vi "Ch_data_title_pattern (SubVI).vi"(9 "Единица измерений":string) -> (0 "error out":errorcluster, 2 "Path":path, 3 "Byte Stream File out":refnum<file>)   [LabVIEW 2015]
panel:
  in  "error in":errorcluster
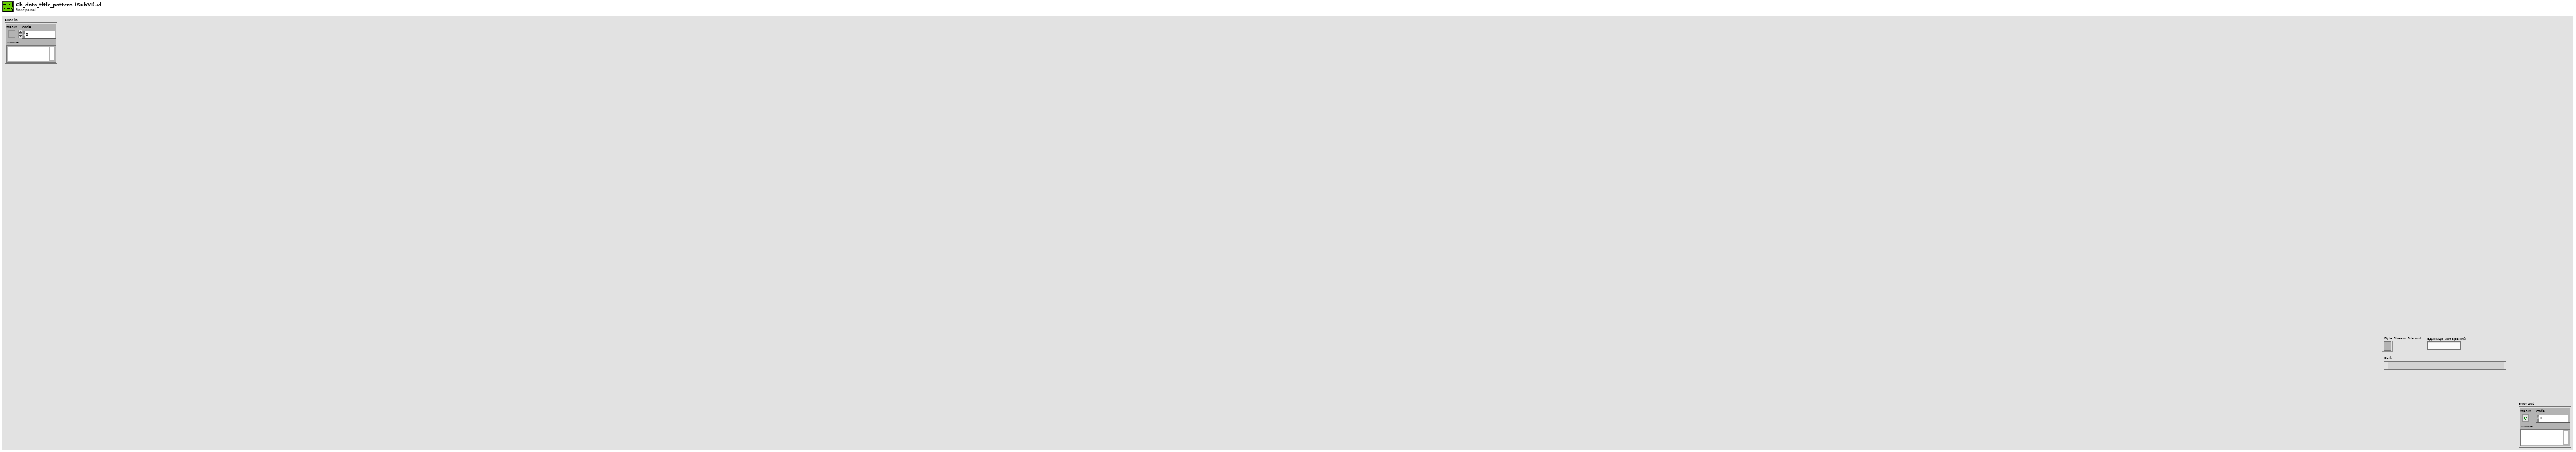
[diagram p1: front panel]
types:
  T1 = enum16{"open", "replace", "create", "open or create", "replace or create", "replace or create with confirmation"}
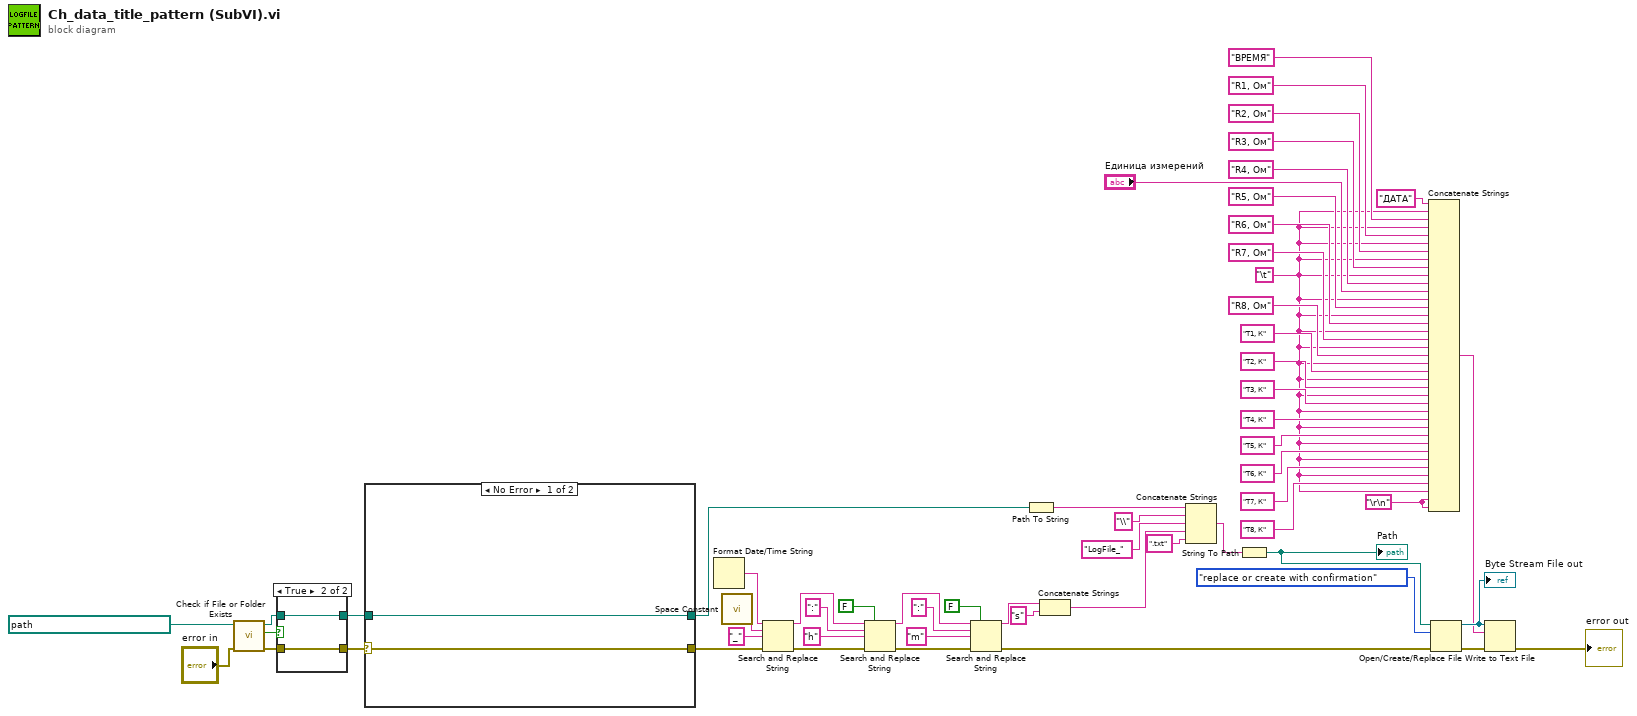
[diagram p0: block diagram]
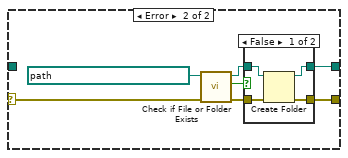
[diagram p2: hidden frame]
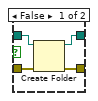
[diagram p4: hidden frame]
diagram:
  w1 = "\t"
  w10 = "\r\n"
  n1 = call <vilib>:"Check if File or Folder Exists.vi"("error in (no error)"="error in", "path"=path "D:/Лог-файл термометрии" ("path (use dialog)")) -> ("error out"=w45:errorcluster, "file or folder exists?"=w43:bool, "dup path"=w46:path)  [unwired: 7 out]
  n2 = case shown="True" w43 {
    tunnel: [w62 w64] -> w41
    tunnel: w46 -> [w61 w64]
    tunnel: w45 -> [w60 w63]
    tunnel: [w59 w63] -> w42
    frame False {
      n3 = Create Folder(path (use dialog)=w61, error in=w60) -> (created path=w62:path, error out=w59:errorcluster)  [unwired: 2 out]
    }
    frame True {
    }
  }
  n4 = case shown="No Error" w42 {
    selector: w42 -> [w65 w67]
    tunnel: w41 -> [w66 _]
    tunnel: [w66 w70] -> w17
    tunnel: [w65 w69] -> w18
    frame No Error {
    }
    frame Error {
      n5 = call <vilib>:"Check if File or Folder Exists.vi"("error in (no error)"=w67, "path"=path "C:/Лог-файл термометрии" ("path (use dialog)")) -> ("error out"=w72:errorcluster, "file or folder exists?"=w71:bool, "dup path"=w73:path)  [unwired: 7 out]
      n6 = case shown="False" w71 {
        tunnel: [w77 w79] -> w70
        tunnel: w73 -> [w76 w79]
        tunnel: w72 -> [w75 w78]
        tunnel: [w74 w78] -> w69
        frame False {
          n7 = Create Folder(path (use dialog)=w76, error in=w75) -> (created path=w77:path, error out=w74:errorcluster)  [unwired: 2 out]
        }
        frame True {
        }
      }
    }
  }
  n8 = Format Date/Time String() -> (date/time string=w39:string)  [unwired: 3 out]
  n9 = call <vilib>:"Space Constant.vi"() -> ("String"=w20:string)
  n10 = Search and Replace String(input string=w39, search string=w20, replace string="_" ("replace string (\"\")"), error in=w18) -> (result string=w22:string, error out=w32:errorcluster)  [unwired: 6 out]
  n11 = Search and Replace String(replace all?=FALSE ("replace all? (F)"), input string=w22, search string=":", replace string="h" ("replace string (\"\")"), error in=w32) -> (result string=w29:string, error out=w33:errorcluster)  [unwired: 5 out]
  n12 = Search and Replace String(replace all?=FALSE ("replace all? (F)"), input string=w29, search string=":", replace string="m" ("replace string (\"\")"), error in=w33) -> (result string=w34:string, error out=w16:errorcluster)  [unwired: 5 out]
  n13 = Path To String(path=w17) -> (string=w30:string)
  n14 = Concatenate Strings(w34, "s" ("string")) -> (w37:string)
  n15 = Concatenate Strings(w30, "\\" ("string"), "LogFile_" ("string"), w37, ".txt" ("default name")) -> (w19:string)
  n16 = String To Path(string=w19) -> (path=w15:path)
  "Path" <- w15
  n17 = Concatenate Strings("ДАТА" ("string"), w1, "ВРЕМЯ" ("string"), w1, "R1, Ом" ("string"), w1, "R2, Ом" ("string"), w1, "R3, Ом" ("string"), w1, "R4, Ом" ("string"), "Единица измерений", w1, "R5, Ом" ("string"), w1, "R6, Ом" ("string"), w1, "R7, Ом" ("string"), w1, "R8, Ом" ("string"), w1, "T1, К" ("string"), w1, "T2, К" ("string"), w1, "T3, К" ("string"), w1, "T4, К" ("string"), w1, "T5, К" ("string"), w1, "T6, К" ("string"), w1, "T7, К" ("string"), w1, "T8, К" ("string"), w1, w10, w10) -> (w49:string)
  n18 = Open/Create/Replace File(file path (use dialog)=w15, error in=w16, operation (0:open)=T1."replace or create with confirmation") -> (refnum out=w52:refnum<file>, error out=w50:errorcluster)  [unwired: 4 out]
  "Byte Stream File out" <- w52
  n19 = Write to Text File(file (use dialog)=w52, text=w49, error in=w50) -> (error out=→"error out":errorcluster)  [unwired: 3 out]
